vi "Add to Tree.vi"(8 "error in (no error)":errorcluster, 9 "Parent Tag":string, 10 "Tree Manager in":refnum<class "Tree Manager.lvclass">, 11 "Attribute in":refnum<class "Attribute.lvclass">) -> (0 "error out":errorcluster, 2 "Tree Manager out":refnum<class "Tree Manager.lvclass">, 3 "Attribute out":refnum<class "Attribute.lvclass">)   [LabVIEW 2018, in "VILab.lvlib" / "Attribute.lvclass"]
uses:
  Attribute.lvclass
  C:/Users/Flarn/Documents/LabVIEW Projects/Low-Level VI Manipulation/Support Files/VILab/Data Item.lvclass
  Tree Manager.lvclass
  Attribute.lvclass/Attribute.ctl
  Data Item.lvclass
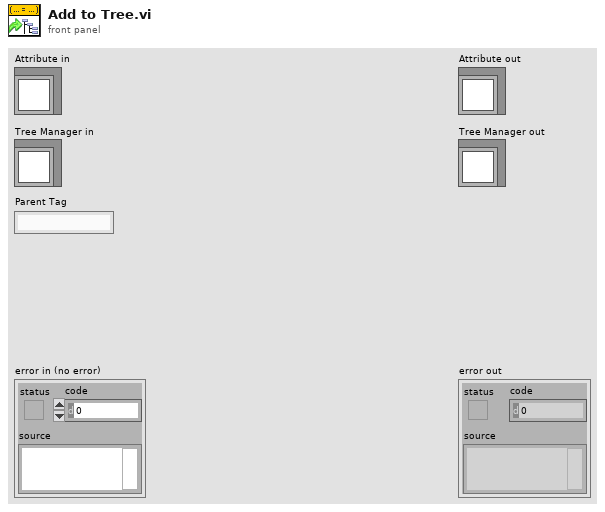
[diagram p1: front panel]
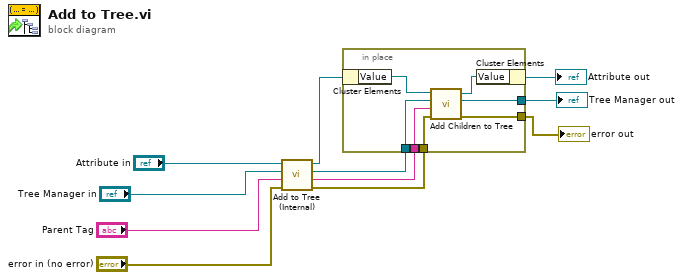
[diagram p0: block diagram]
diagram:
  n1 = call "Add to Tree (Internal).vi"("error in (no error)"="error in (no error)", "Parent Tag"="Parent Tag", "Tree Manager in"="Tree Manager in", "Data Item in"="Attribute in") -> ("error out"=w6:errorcluster, "New Tag"=w4:string, "Tree Manager out"=w5:refnum<class "Tree Manager.lvclass">, "Data Item out"=w7:refnum<class "Attribute.lvclass">)  [unwired: 4 in]
  n2 = in-place {
    in-place-border: w6 -> [w16]
    in-place-border: w5 -> [w15]
    in-place-border: w4 -> [w14]
    in-place-border: [w13] -> w2
    in-place-border: [w12] -> w1
    n3 = in-place-cluster #1(w7) -> ("Value"=w18:refnum<class "Data Item.lvclass">)
    n4 = call "Add Children to Tree.vi"("error in (no error)"=w16, "Parent Tag"=w14, "Tree Manager in"=w15, "Data Item in"=w18) -> ("error out"=w12:errorcluster, "Tree Manager out"=w13:refnum<class "Tree Manager.lvclass">, "Data Item out"=w17:refnum<class "Data Item.lvclass">)  [unwired: 5 in]
    n5 = in-place-cluster #1("Value"=w17) -> (→"Attribute out":refnum<class "Attribute.lvclass">)
  }
  "error out" <- w1
  "Tree Manager out" <- w2
